vi "rename channel test.vi"() -> ()   [LabVIEW 2013, in "tag select module tests.lvlib"]
uses:
  tag select module tests.lvlib
  module/configuration/tag select configuration.ctl
  <vilib>/NI/Tag Bus Module Framework/channel/TBM channel.lvclass
  <vilib>/NI/Tag Bus/tag/Data Type.ctl
  module/configuration/tag select module configuration.lvclass/tag select module configuration.ctl
  <vilib>/NI/Tag Bus/tag/tag descriptor.lvclass/tag descriptor.ctl
  module/configuration/Read tag select.vi
  module/configuration/tag select module configuration.lvclass
  <vilib>/NI/Tag Bus/tag/tag descriptor.lvclass
panel:
  out "data Input B 2":T1
  out "data input A 2":T1
  out "data select 2":T1
  out "data output 2":T1
  out "data Input B":T1
  out "data input A":T1
  out "data select":T1
  out "data output":T1
  out "input B 2":string
  out "input A 2":string
  out "input B":string
  out "input A":string
  out "select 2":string
  out "output 2":string
  out "select":string
  out "output":string
  out "tag select 2":T2[](array[typedef])
  out "tag select":T2[](array[typedef])
  out "no err":errorcluster
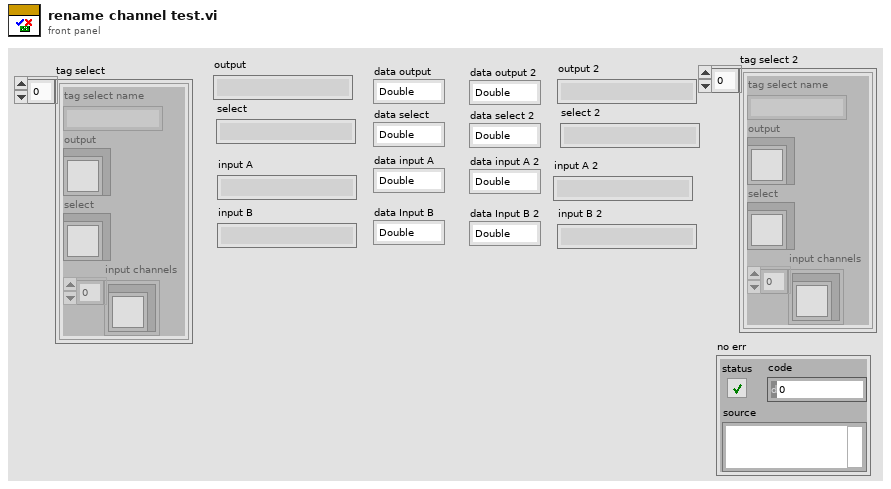
[diagram p1: front panel]
types:
  T1 = typedef "tag bus.lvlib/tag descriptor.lvclass/Data Type.ctl" = enum16{"Double", "Single", "I64", "I32", "I16", "I8", "U64", "U32", "U16", "U8", "Boolean", "String", "Array of Double", "Array of Single", "Array of I64", "Array of I32", "Array of I16", "Array of I8", "Array of U64", "Array of U32", "Array of U16", "Array of U8", "Array of Boolean", "Array of String"}
  T2 = typedef "tag select module configuration.lvclass/tag select configuration.ctl" = cluster{"tag select name":string, "output":refnum<class "TBM channel.lvclass">, "select":refnum<class "TBM channel.lvclass">, "input channels":refnum<class "TBM channel.lvclass">[]}
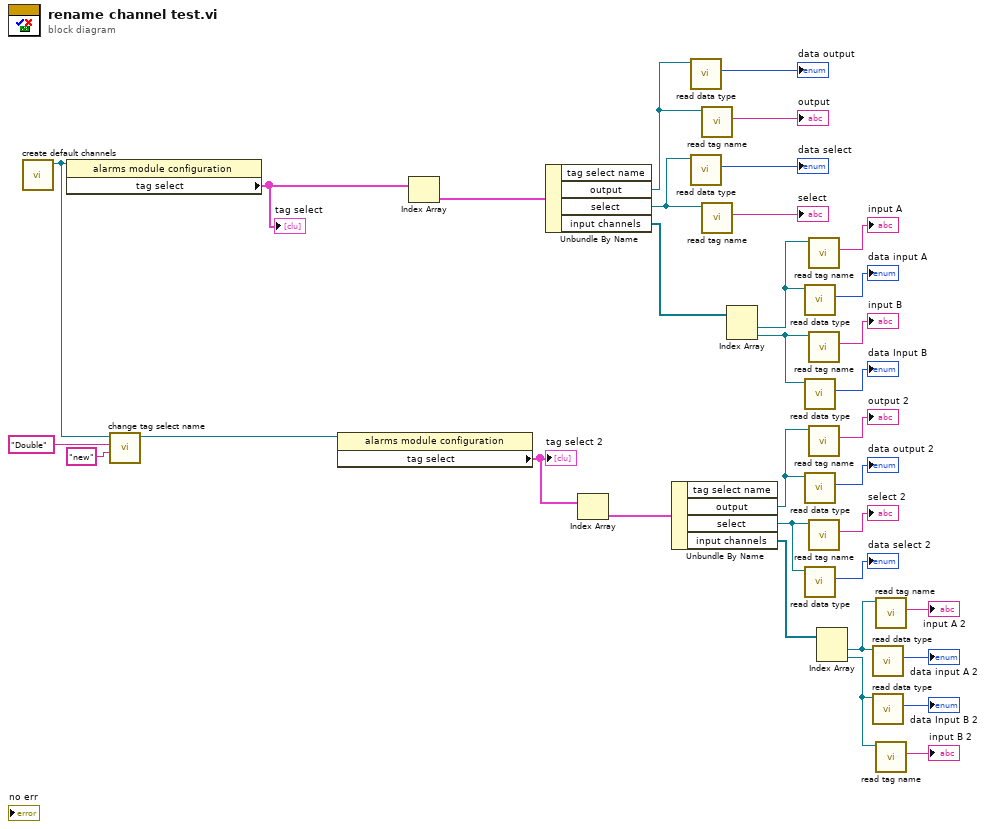
[diagram p0: block diagram]
diagram:
  n1 = call "create default channels.vi"() -> ("module"=w32:refnum<class "tag select module configuration.lvclass">)  [unwired: 8 in, 3 out]
  n2 = property class="alarms module configuration"(reference=w32) -> ("tag select"=w30:T2[])  [unwired: 1 in, 2 out]
  "tag select" <- w30
  n3 = call "change tag select name.vi"("new name"="new", "old name"="Double", "tag select module configuration in"=w32) -> ("tag select module configuration out"=w31:refnum<class "tag select module configuration.lvclass">)  [unwired: 6 in, 2 out]
  n4 = property class="alarms module configuration"(reference=w31) -> ("tag select"=w23:T2[])  [unwired: 1 in, 2 out]
  "tag select 2" <- w23
  n5 = Index Array(array=w30) -> (element=w29:T2)  [unwired: 1 in]
  n6 = Unbundle By Name(w29) -> ("output"=w9:refnum<class "TBM channel.lvclass">, "select"=w10:refnum<class "TBM channel.lvclass">, "input channels"=w22:refnum<class "TBM channel.lvclass">[])  [unwired: 1 out]
  n7 = Index Array(array=w23) -> (element=w26:T2)  [unwired: 1 in]
  n8 = Unbundle By Name(w26) -> ("output"=w4:refnum<class "TBM channel.lvclass">, "select"=w3:refnum<class "TBM channel.lvclass">, "input channels"=w17:refnum<class "TBM channel.lvclass">[])  [unwired: 1 out]
  n9 = call <vilib>:"read data type.vi"("system tag in"=w9) -> ("data type"=→"data output":T1)  [unwired: 8 in, 2 out]
  n10 = call <vilib>:"read data type.vi"("system tag in"=w10) -> ("data type"=→"data select":T1)  [unwired: 8 in, 2 out]
  n11 = call <vilib>:"read tag name.vi"("system tag in"=w9) -> ("name"=→"output":string)  [unwired: 8 in, 2 out]
  n12 = call <vilib>:"read tag name.vi"("system tag in"=w10) -> ("name"=→"select":string)  [unwired: 8 in, 2 out]
  n13 = Index Array(array=w22) -> (element #1=w11:refnum<class "TBM channel.lvclass">, element #2=w12:refnum<class "TBM channel.lvclass">)  [unwired: 2 in]
  n14 = call <vilib>:"read data type.vi"("system tag in"=w11) -> ("data type"=→"data input A":T1)  [unwired: 8 in, 2 out]
  n15 = call <vilib>:"read data type.vi"("system tag in"=w12) -> ("data type"=→"data Input B":T1)  [unwired: 8 in, 2 out]
  n16 = call <vilib>:"read data type.vi"("system tag in"=w4) -> ("data type"=→"data output 2":T1)  [unwired: 8 in, 2 out]
  n17 = call <vilib>:"read data type.vi"("system tag in"=w3) -> ("data type"=→"data select 2":T1)  [unwired: 8 in, 2 out]
  n18 = call <vilib>:"read tag name.vi"("system tag in"=w11) -> ("name"=→"input A":string)  [unwired: 8 in, 2 out]
  n19 = call <vilib>:"read tag name.vi"("system tag in"=w12) -> ("name"=→"input B":string)  [unwired: 8 in, 2 out]
  n20 = call <vilib>:"read tag name.vi"("system tag in"=w4) -> ("name"=→"output 2":string)  [unwired: 8 in, 2 out]
  n21 = call <vilib>:"read tag name.vi"("system tag in"=w3) -> ("name"=→"select 2":string)  [unwired: 8 in, 2 out]
  n22 = Index Array(array=w17) -> (element #1=w2:refnum<class "TBM channel.lvclass">, element #2=w1:refnum<class "TBM channel.lvclass">)  [unwired: 2 in]
  n23 = call <vilib>:"read data type.vi"("system tag in"=w2) -> ("data type"=→"data input A 2":T1)  [unwired: 8 in, 2 out]
  n24 = call <vilib>:"read data type.vi"("system tag in"=w1) -> ("data type"=→"data Input B 2":T1)  [unwired: 8 in, 2 out]
  n25 = call <vilib>:"read tag name.vi"("system tag in"=w2) -> ("name"=→"input A 2":string)  [unwired: 8 in, 2 out]
  n26 = call <vilib>:"read tag name.vi"("system tag in"=w1) -> ("name"=→"input B 2":string)  [unwired: 8 in, 2 out]
